vi "Create.vi"(0 "ClassWriterGOOP300.lvclass":refnum<class "ClassWriterGOOP300.lvclass">, 5 "error in (no error)":errorcluster) -> (14 "ClassWriterGOOP300.lvclass":refnum<class "ClassWriterGOOP300.lvclass">, 19 "error out":errorcluster)   [LabVIEW 2020, in "ClassWriterGOOP300.lvclass"]
uses:
  <resource>/Framework/Providers/Open_GDS/ClassProviders/Provider_EndevoGOOP300/ClassWriterGOOP300_class/ClassWriterGOOP300.lvclass
  <resource>/Framework/Providers/Open_GDS/ClassProviders/Provider_LvNativeClass/ClassWriterNative_class/ClassWriterNative.lvclass
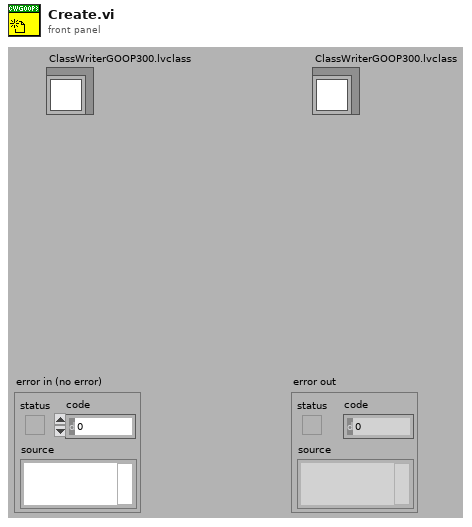
[diagram p1: front panel]
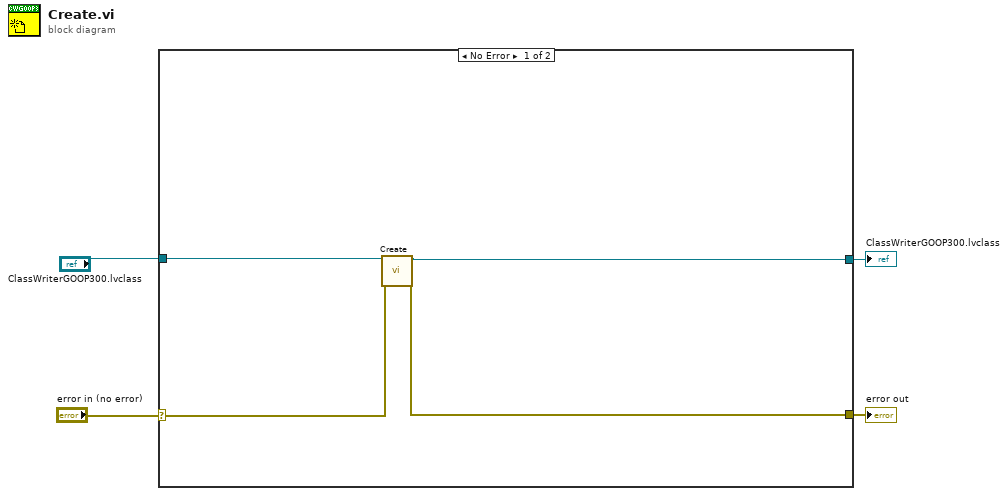
[diagram p0: block diagram]
diagram:
  n1 = case shown="No Error" "error in (no error)" {
    selector: "error in (no error)" -> [w7 w10]
    tunnel: [w5 w9] -> w4
    tunnel: [w6 w10] -> w3
    tunnel: "ClassWriterGOOP300.lvclass" -> [w8 w9]
    frame No Error {
      n2 = call-parent "Create.vi"("ClassWriterNative"=w8, "error in (no error)"=w7) -> ("ClassWriterNative"=w5:refnum<class "ClassWriterGOOP300.lvclass">, "error out"=w6:errorcluster)  [unwired: 16 in]
    }
    frame Error {
    }
  }
  "error out" <- w3
  "ClassWriterGOOP300.lvclass" <- w4
